vi "StringToGFG.vi"(9 "Source VI":string, 10 "VariableValueString":string, 11 "Variable Name In":string) -> ()   [LabVIEW 2012]
doc: "SciScan 1.2 160622"
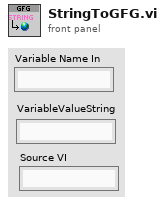
[diagram p1: front panel]
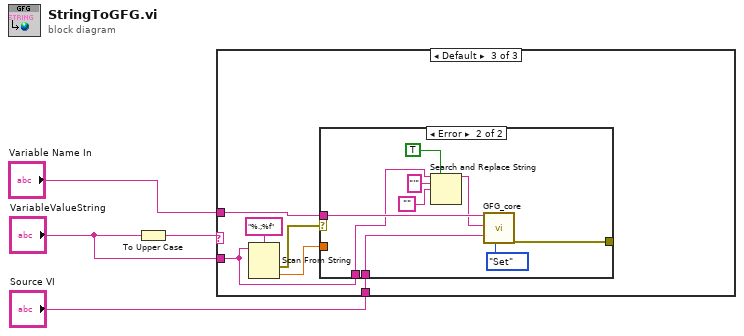
[diagram p0: block diagram]
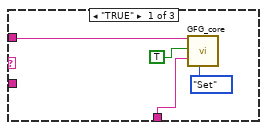
[diagram p2: hidden frame]
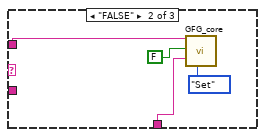
[diagram p3: hidden frame]
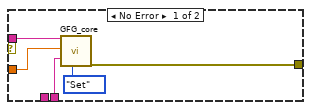
[diagram p4: hidden frame]
diagram:
  n1 = To Upper Case(1:"VariableValueString") -> (0:w2:string)
  n2 = case shown="Default" w2 {
    tunnel: "Variable Name In" -> [w8 w12 w18]
    tunnel: "Source VI" -> [w5 w9 w14]
    tunnel: "VariableValueString" -> [_ _ w13]
    frame "TRUE" {
      n3 = call "GFG_core.vi"("Variable Name in"=w8, "Variant in"=TRUE, "Source VI"=w5, "Action"=enum16{"Init", "Set", "Get"}."Set") -> ()  [unwired: 9 in, 7 out]
    }
    frame "FALSE" {
      n4 = call "GFG_core.vi"("Variable Name in"=w12, "Variant in"=FALSE, "Source VI"=w9, "Action"=enum16{"Init", "Set", "Get"}."Set") -> ()  [unwired: 9 in, 7 out]
    }
    frame Default {
      n5 = Scan From String(format string="%.;%f" ("Format String"), input string=w13) -> (error out=w16:errorcluster, output 1=w15:dbl)  [unwired: 3 in, 2 out]
      n6 = case shown="Error" w16 {
        tunnel: w18 -> [w23 w32]
        tunnel: [w21 w30] -> _
        tunnel: w15 -> [w20 _]
        tunnel: w13 -> [_ w25]
        tunnel: w14 -> [w19 w26]
        frame No Error {
          n7 = call "GFG_core.vi"("Variable Name in"=w23, "Variant in"=w20, "Source VI"=w19, "Action"=enum16{"Init", "Set", "Get"}."Set") -> ("error out"=w21:errorcluster)  [unwired: 9 in, 6 out]
        }
        frame Error {
          n8 = Search and Replace String(replace all?=TRUE ("replace all? (F)"), input string=w25, search string="'", replace string="") -> (result string=w24:string)  [unwired: 4 in, 3 out]
          n9 = call "GFG_core.vi"("Variable Name in"=w32, "Variant in"=w24, "Source VI"=w26, "Action"=enum16{"Init", "Set", "Get"}."Set") -> ("error out"=w30:errorcluster)  [unwired: 9 in, 6 out]
        }
      }
    }
  }
